vi "Type to String.vi"() -> ()   [LabVIEW 2015]
uses:
  <vilib>/Utility/error.llb/DialogType.ctl
  source/library/Scripting.lvlib
  <vilib>/LV-Scripting/LV-Scripting.lvlib
  <vilib>/Utility/Data Type/NI_Data Type.lvlib
panel:
  out "Element Types":variant[](array[variant])
  out "length":i32
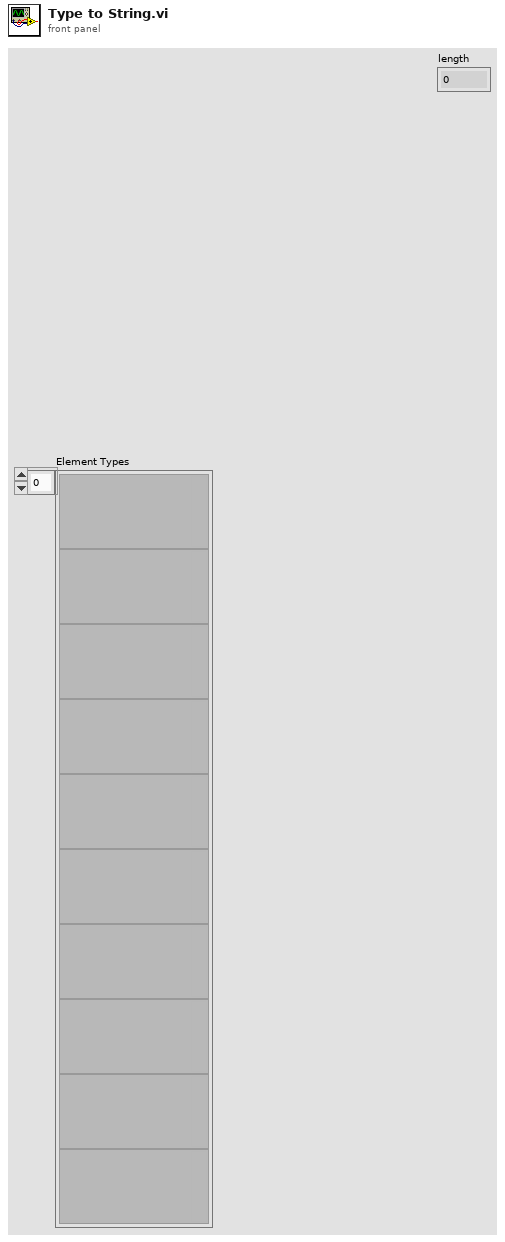
[diagram p1: front panel]
types:
  T1 = typedef "DialogType.ctl" = u16
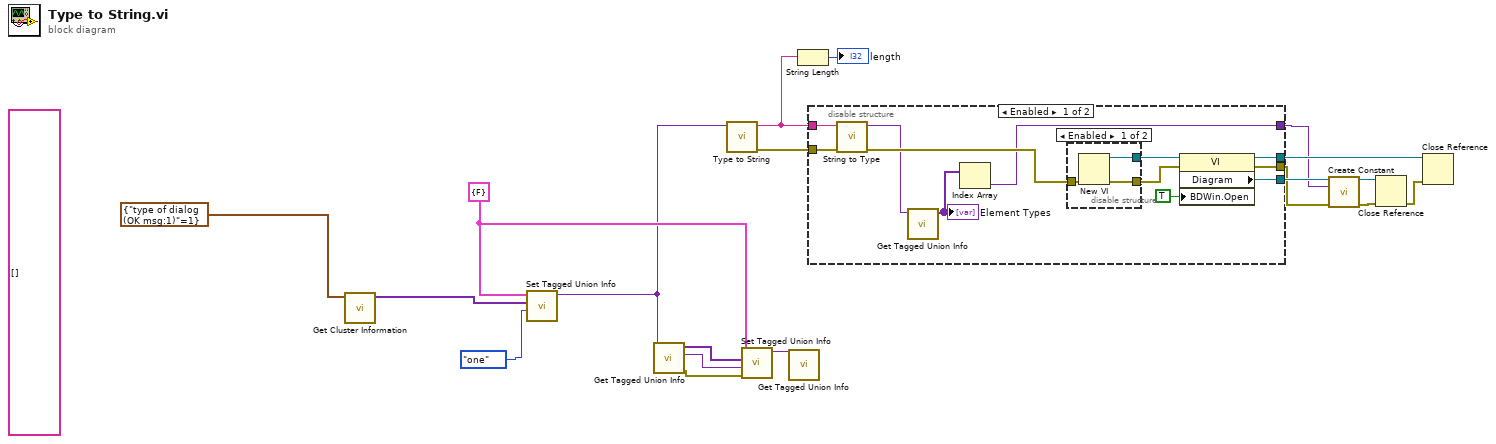
[diagram p0: block diagram]
diagram:
  (unwired) string[][][][][][][][][][][][][][][][][][][] []
  w2 = cluster{bool} {FALSE}
  n1 = call <vilib>:"Get Cluster Information.vi"("Variant"=cluster{"type of dialog (OK msg:1)":T1} {"type of dialog (OK msg:1)"=1}) -> ("Cluster Elements"=w3:variant[])  [unwired: 9 in, 1 out]
  n2 = call "Set Tagged Union Info.vi"("Enum Type"=enum16{"one"}."one", "Element Types"=w3, "Variant in"=w2) -> ("Variant out"=w1:variant)  [unwired: 7 in, 1 out]
  n3 = call "Get Tagged Union Info.vi"("Type in"=w1) -> ("error out"=w9:errorcluster, "Enum Type"=w4:variant, "Element Types"=w8:variant[])  [unwired: 8 in]
  n4 = call "Type to String.vi"("Type"=w1) -> ("Error Out"=w19:errorcluster, "String"=w11:string)  [unwired: 9 in]
  n5 = call "Set Tagged Union Info.vi"("error in (no error)"=w9, "Enum Type"=w4, "Element Types"=w8, "Variant in"=w2) -> ("Variant out"=w7:variant)  [unwired: 6 in, 1 out]
  n6 = call "Get Tagged Union Info.vi"("Type in"=w7) -> ()  [unwired: 8 in, 3 out]
  n7 = String Length(string=w11) -> (length=→"length":i32)
  n8 = disable-structure shown="Enabled" {
    disable-tunnel: w19 -> [w31 _]
    disable-tunnel: [w30 _] -> w17
    disable-tunnel: [w29 _] -> w16
    disable-tunnel: [w28 _] -> w12
    disable-tunnel: [w20 _] -> w6
    disable-tunnel: w11 -> [w27 _]
    frame Enabled {
      n9 = call "String to Type.vi"("Error In"=w31, "String"=w27) -> ("Error Out"=w26:errorcluster, "Type"=w21:variant)  [unwired: 7 in, 1 out]
      n10 = call "Get Tagged Union Info.vi"("Type in"=w21) -> ("Element Types"=w22:variant[])  [unwired: 8 in, 2 out]
      "Element Types" <- w22
      n11 = Index Array(array=w22) -> (element=w20:variant)  [unwired: 1 in]
      n12 = disable-structure shown="Enabled" {
        disable-tunnel: w26 -> [w34 _]
        disable-tunnel: [w33 _] -> w25
        disable-tunnel: [w32 _] -> w23
        frame Enabled {
          n13 = New VI(8:w34) -> (0:w32:errorcluster, 3:w33:refnum<vi>)  [unwired: 6 in]
        }
        frame Disabled {
        }
      }
      n14 = property class="VI"(reference=w25, error in=w23, "BDWin.Open"=TRUE ("Block Diagram Window:Open")) -> (reference out=w28:refnum<vi>, error out=w29:errorcluster, "Diagram"=w30:refnum<vi>)
    }
    frame Disabled {
    }
  }
  n15 = call <vilib>:"Create Constant.vi"("Diagram in"=w17, "Type"=w6, "error in (no error)"=w16) -> ("Diagram out"=w14:refnum<vi>, "error out"=w15:errorcluster)  [unwired: 10 in, 1 out]
  n16 = Close Reference(reference=w14, error in (no error)=w15) -> (error out=w13:errorcluster)
  n17 = Close Reference(reference=w12, error in (no error)=w13) -> ()  [unwired: 1 out]
